vi "CIA1_IRQ.vi"(7 "oper":T1, 10 "IRQ flag idx":u8, 11 "Dx0E value":u8 format="%02x") -> (1 "IRQ.active":bool, 2 "IRQ.reg":u8 format="%08b")   [LabVIEW 2018]
uses:
  CIA_IRQ_oper.ctl
  CIA1_glb.vi
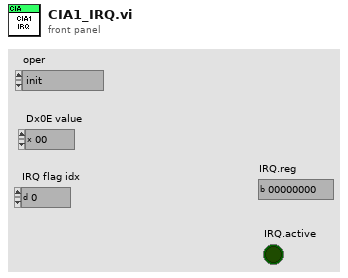
[diagram p1: front panel]
types:
  T1 = typedef "CIA_IRQ_oper.ctl" = enum16{"init", "set mask", "set flag", "check active", "read reg"}
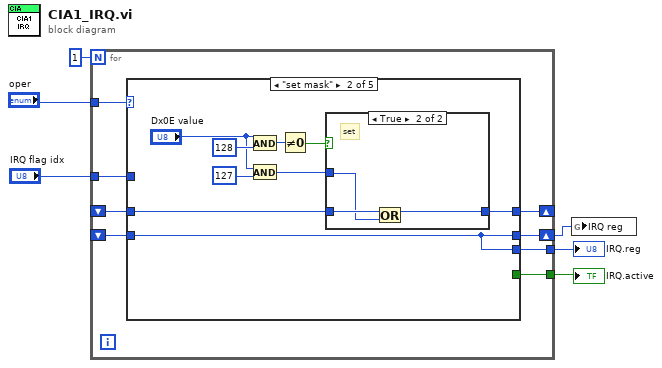
[diagram p0: block diagram]
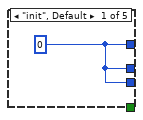
[diagram p2: hidden frame]
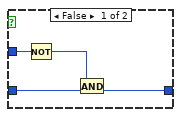
[diagram p3: hidden frame]
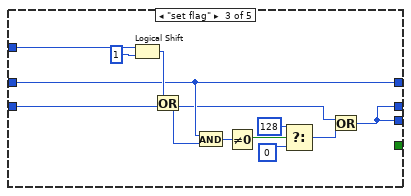
[diagram p4: hidden frame]
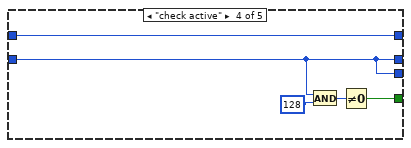
[diagram p5: hidden frame]
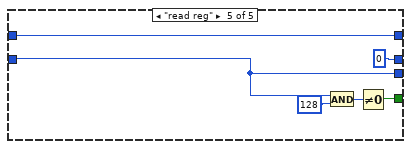
[diagram p6: hidden frame]
diagram:
  n1 = for {
    N: 1 -> [_]
    shift-right: [w13] -> _
    shift-left: _ -> [w12]
    tunnel: "oper" -> [w14]
    shift-right: [w8] -> w1
    shift-left: _ -> [w11]
    tunnel: "IRQ flag idx" -> [w10]
    tunnel: [w9] -> w3
    tunnel: [w7] -> w2
    n2 = case shown="\"set mask\"" w14 {
      tunnel: [w15 w18 w39 w45 w54] -> w13
      tunnel: w12 -> [_ w20 w39 w45 w54]
      tunnel: w11 -> [_ w17 w41 w44 w49]
      tunnel: [w15 w17 w32 w44 u8 0 ("mask")] -> w8
      tunnel: w10 -> [_ _ w42 _ _]
      tunnel: [_ _ _ w48 w50] -> w9
      tunnel: [w15 w17 w32 w44 w49] -> w7
      frame "init", Default {
        w15 = u8 0 ("mask")
      }
      frame "set mask" {
        n3 = And(x="Dx0E value", y=u8 128) -> (x .and. y?=w23:u8)
        n4 = And(x="Dx0E value", y=u8 127) -> (x .and. y?=w19:u8)
        n5 = Not Equal To 0?(x=w23) -> (x != 0?=w21:bool)
        n6 = case shown="True" w21 {
          tunnel: w20 -> [w26 w31]
          tunnel: w19 -> [w28 w30]
          tunnel: [w25 w29] -> w18
          frame False {
            n7 = Not(x=w28) -> (.not. x?=w27:u8)
            n8 = And(x=w27, y=w26) -> (x .and. y?=w25:u8)
          }
          frame True {
            # "set"
            n9 = Or(x=w31, y=w30) -> (x .or. y?=w29:u8)
          }
        }
      }
      frame "set flag" {
        n10 = Logical Shift(y=w42, x=u8 1) -> (x << y=w40:u8)
        n11 = Or(x=w40, y=w41) -> (x .or. y?=w33:u8)
        n12 = And(x=w39, y=w33) -> (x .and. y?=w38:u8)
        n13 = Not Equal To 0?(x=w38) -> (x != 0?=w37:bool)
        n14 = Select(t=u8 128 ("x"), s=w37, f=u8 0 ("x")) -> (s? t:f=w34:u8)
        n15 = Or(x=w33, y=w34) -> (x .or. y?=w32:u8)
      }
      frame "check active" {
        n16 = And(x=w44, y=u8 128) -> (x .and. y?=w46:u8)
        n17 = Not Equal To 0?(x=w46) -> (x != 0?=w48:bool)
      }
      frame "read reg" {
        n18 = And(x=w49, y=u8 128) -> (x .and. y?=w51:u8)
        n19 = Not Equal To 0?(x=w51) -> (x != 0?=w50:bool)
      }
    }
  }
  "IRQ.reg" <- w2
  "IRQ.active" <- w3
  n20 = global write "CIA1_glb.vi" "IRQ reg"(w1) -> ()
